vi "DAQ Control_Start_Switch.vi"(3 "error in":errorcluster, 5 "task in":refnum<k21>) -> (0 "Data":bool, 1 "error out":errorcluster, 2 "task out":refnum<k21>)   [LabVIEW 2023]
uses:
  <vilib>/DAQmx/miscellaneous.llb/DAQmx Fill In Error Info.vi
  <vilib>/DAQmx/read.llb/DAQmx Read (Digital Bool 1Line 1Point).vi
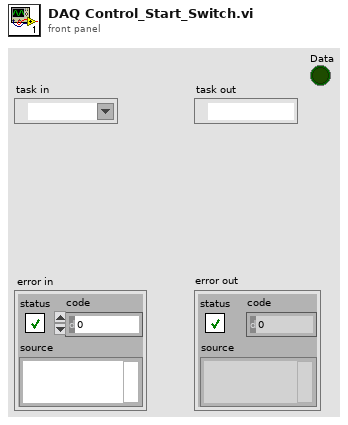
[diagram p1: front panel]
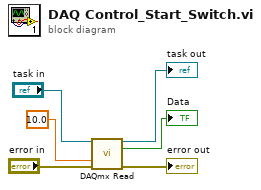
[diagram p0: block diagram]
diagram:
  n1 = call-poly <vilib>:"DAQmx Read.vi"("task/channels in"="task in", "timeout"=10.0, "error in"="error in") -> ("task out"=→"task out":refnum<k21>, "data"=→"Data":bool, "error out"=→"error out":errorcluster)  [unwired: 10 in]
